vi "Autonomous Independent.vi"() -> (3 "LED ms toggle rate":u32=500)   [LabVIEW 2013]
doc: "This VI is called when autonomous begins, and will automatically be terminated when autonomous ends. You can carry out timed or sensor driven robot movement independently without needing to return to the caller."
uses:
  Robot Global Data.vi
panel:
  out "Distance":dbl
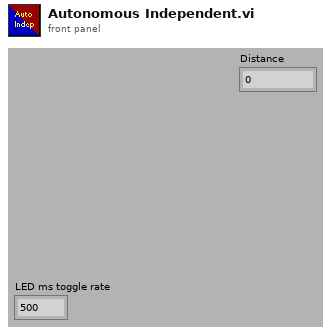
[diagram p1: front panel]
types:
  T1 = typedef "WPI_EncoderDevRef.ctl" = cluster{"DevStatus":errorcluster, "EncoderIndex":T2, "CounterIndex":T3, "DistancePerCount":dbl, "Decoding Type":T4}
  T2 = typedef "FPGA_EncoderIdx.ctl" = enum8{"Enc 0", "Enc 1", "Enc 2", "Enc 3", "Invalid"}
  T3 = typedef "FPGA_CounterCtrSystemIndex.ctl" = enum8{"Ctr 0", "Ctr 1", "Ctr 2", "Ctr 3", "Ctr 4", "Ctr 5", "Ctr 6", "Ctr 7", "Invalid"}
  T4 = typedef "WPI_EncoderType.ctl" = enum16{"1x", "2x", "4x"}
  T5 = typedef "WPI_MotorControlDeviceRef.ctl" = cluster{"DeviceStatus":errorcluster, "Type":enum16{"PWM", "CAN"}, "PWM":cluster{"Digital Module":T6, "PWM Channel":T7, "DeadBand":T8}, "CAN":cluster{"Device Number":u8, "Control Mode":T9, "Semaphore":T10, "Max Vout":dbl}, "Invert":bool, "TransformRef":T11, "InvTransformRef":T11}
  T6 = typedef "FPGA_TypedefDigitalModule.ctl" = enum16{"Digital Module 1", "Digital Module 2"}
  T7 = typedef "FPGA_DIOPWMChannel.ctl" = enum8{"PWM 1", "PWM 2", "PWM 3", "PWM 4", "PWM 5", "PWM 6", "PWM 7", "PWM 8", "PWM 9", "PWM 10", "Invalid"}
  T8 = typedef "WPI_PWMDeadband.ctl" = cluster{"Name":string, "maxPositivePwm":i32, "minPositivePwm":i32, "centerPwm":i32, "maxNegativePwm":i32, "minNegativePwm":i32, "angularRange":u16}
  T9 = typedef "WPI_CANJaguar_ControlMode.ctl" = enum8{"Percent VBus", "Current", "Speed", "Position", "Voltage"}
  T10 = typedef "Semaphore RefNum" = refnum<k1>
  T11 = typedef "WPI_PWMTransform_ConPane.ctl" = refnum<vi>
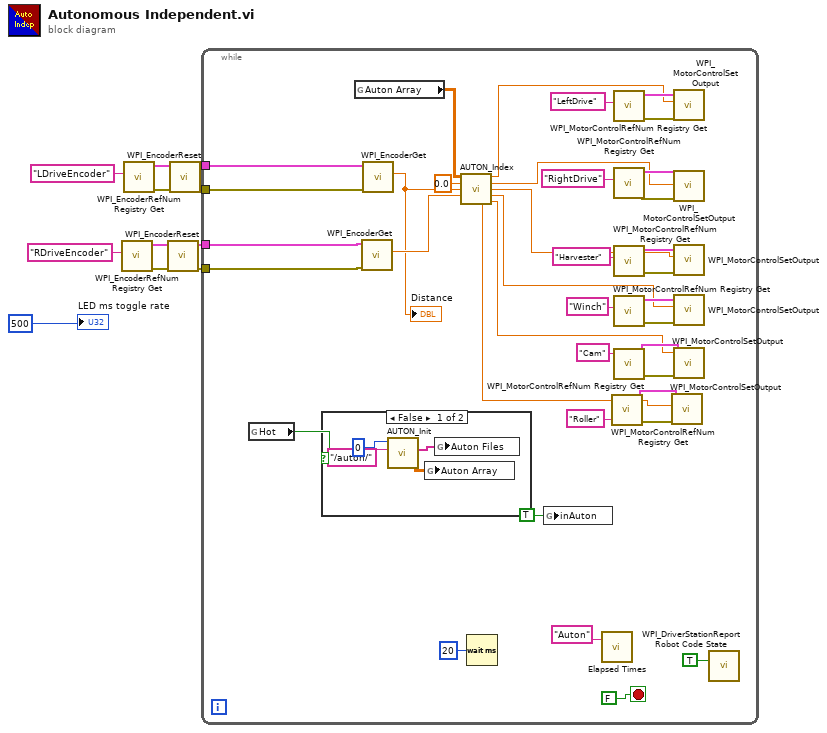
[diagram p0: block diagram]
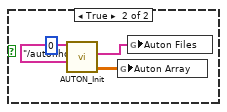
[diagram p2: hidden frame]
diagram:
  n1 = call <vilib>:"WPI_EncoderRefNum Registry Get.vi"("refnum name"="RDriveEncoder") -> ("error out"=w3:errorcluster, "EncoderDevRef"=w5:T1)  [unwired: 9 in]
  n2 = call <vilib>:"WPI_EncoderRefNum Registry Get.vi"("refnum name"="LDriveEncoder") -> ("error out"=w9:errorcluster, "EncoderDevRef"=w8:T1)  [unwired: 9 in]
  n3 = call <vilib>:"WPI_EncoderReset.vi"("error in (no error)"=w3, "EncoderDevRef"=w5) -> ("error out"=w1:errorcluster, "EncoderDevRef"=w2:T1)  [unwired: 8 in]
  n4 = call <vilib>:"WPI_EncoderReset.vi"("error in (no error)"=w9, "EncoderDevRef"=w8) -> ("error out"=w6:errorcluster, "EncoderDevRef"=w7:T1)  [unwired: 8 in]
  n5 = while {
    tunnel: w7 -> [w47]
    tunnel: w6 -> [w46]
    tunnel: w2 -> [w44]
    tunnel: w1 -> [w43]
    stop <- FALSE stop-if-true
    n6 = global read "Robot Global Data.vi" "Hot"() -> (w12:bool)
    n7 = case shown="False" w12 {
      frame False {
        n8 = call "AUTON_Init.vi"("Directory"="/auton/", "Default File"=0) -> ("Auton Array"=w52:dbl[][], "Auton Files"=w51:string[])  [unwired: 7 in, 1 out]
        n9 = global write "Robot Global Data.vi" "Auton Array"(w52) -> ()
        n10 = global write "Robot Global Data.vi" "Auton Files"(w51) -> ()
      }
      frame True {
        n11 = call "AUTON_Init.vi"("Directory"="/autonhot/", "Default File"=0) -> ("Auton Array"=w56:dbl[][], "Auton Files"=w55:string[])  [unwired: 7 in, 1 out]
        n12 = global write "Robot Global Data.vi" "Auton Array"(w56) -> ()
        n13 = global write "Robot Global Data.vi" "Auton Files"(w55) -> ()
      }
    }
    n14 = global read "Robot Global Data.vi" "Auton Array"() -> (w22:dbl[][])
    n15 = call <vilib>:"WPI_EncoderGet.vi"("error in (no error)"=w43, "EncoderDevRef"=w44) -> ("Distance"=w42:dbl)  [unwired: 4 in, 5 out]
    n16 = call <vilib>:"WPI_EncoderGet.vi"("error in (no error)"=w46, "EncoderDevRef"=w47) -> ("Distance"=w16:dbl)  [unwired: 4 in, 5 out]
    "Distance" <- w16
    n17 = call "AUTON_Index.vi"("Auton Array"=w22, "MeasuredHeading"=0.0, "LeftEncoder"=w16, "RightEncoder"=w42) -> ("Right Drive"=w23:dbl, "Left Drive"=w13:dbl, "Harvester"=w32:dbl, "Winch"=w25:dbl, "Roller"=w18:dbl, "Cam"=w24:dbl)  [unwired: 6 in]
    n18 = Wait (ms)(milliseconds to wait=u32 20) -> ()  [unwired: 1 out]
    n19 = global write "Robot Global Data.vi" "inAuton"(TRUE ("inAuton")) -> ()
    n20 = call "Elapsed Times.vi"("Call Name"="Auton") -> ()  [unwired: 2 in, 1 out]
    n21 = call <vilib>:"WPI_MotorControlRefNum Registry Get.vi"("refnum name"="Roller") -> ("error out"=w20:errorcluster, "MotorControlDevRef"=w21:T5)  [unwired: 9 in]
    n22 = call <vilib>:"WPI_MotorControlRefNum Registry Get.vi"("refnum name"="LeftDrive") -> ("error out"=w37:errorcluster, "MotorControlDevRef"=w38:T5)  [unwired: 9 in]
    n23 = call <vilib>:"WPI_MotorControlRefNum Registry Get.vi"("refnum name"="RightDrive") -> ("error out"=w33:errorcluster, "MotorControlDevRef"=w34:T5)  [unwired: 9 in]
    n24 = call <vilib>:"WPI_MotorControlRefNum Registry Get.vi"("refnum name"="Harvester") -> ("error out"=w35:errorcluster, "MotorControlDevRef"=w36:T5)  [unwired: 9 in]
    n25 = call <vilib>:"WPI_MotorControlRefNum Registry Get.vi"("refnum name"="Winch") -> ("error out"=w31:errorcluster, "MotorControlDevRef"=w27:T5)  [unwired: 9 in]
    n26 = call <vilib>:"WPI_MotorControlRefNum Registry Get.vi"("refnum name"="Cam") -> ("error out"=w28:errorcluster, "MotorControlDevRef"=w26:T5)  [unwired: 9 in]
    n27 = call <vilib>:"WPI_MotorControlSetOutput.vi"("error in (no error)"=w20, "Output"=w18, "MotorControlDevRef"=w21) -> ()  [unwired: 6 in, 3 out]
    n28 = call <vilib>:"WPI_MotorControlSetOutput.vi"("error in (no error)"=w37, "Output"=w23, "MotorControlDevRef"=w38) -> ()  [unwired: 6 in, 3 out]
    n29 = call <vilib>:"WPI_MotorControlSetOutput.vi"("error in (no error)"=w33, "Output"=w13, "MotorControlDevRef"=w34) -> ()  [unwired: 6 in, 3 out]
    n30 = call <vilib>:"WPI_MotorControlSetOutput.vi"("error in (no error)"=w35, "Output"=w32, "MotorControlDevRef"=w36) -> ()  [unwired: 6 in, 3 out]
    n31 = call <vilib>:"WPI_MotorControlSetOutput.vi"("error in (no error)"=w31, "Output"=w25, "MotorControlDevRef"=w27) -> ()  [unwired: 6 in, 3 out]
    n32 = call <vilib>:"WPI_MotorControlSetOutput.vi"("error in (no error)"=w28, "Output"=w24, "MotorControlDevRef"=w26) -> ()  [unwired: 6 in, 3 out]
    n33 = call <vilib>:"WPI_DriverStationReport Robot Code State.vi"("Autonomous"=TRUE) -> ()  [unwired: 10 in, 1 out]
  }
  "LED ms toggle rate" <- u32 500 ("LED ms toggle rate")
